vi "Main Tclk.vi"() -> ()   [LabVIEW 2018] (continued)
                            }
                          }
                          n5159 = Select(t="^delete" ("replace string (\"\")"), s=w4601, f="^keep" ("replace string (\"\")")) -> (s? t:f=w4605:string)
                          n5160 = Search and Replace String(input string=w4610, search string=":", replace string=w4611) -> (result string=w4607:string)  [unwired: 5 in, 3 out]
                          n5161 = Concatenate Strings(w4602, "^" ("string"), w4607, w4605) -> (w4616:string)
                          n5162 = Build Path(base path=w4615, name or relative path=w4616) -> (appended path=w4617:path)
                          n5163 = Open/Create/Replace File(file path (use dialog)=w4617, operation (0:open)=T49."replace or create") -> (refnum out=w4620:refnum<file>, error out=w4622:errorcluster)  [unwired: 1 in, 4 out]
                          n5164 = Close File(refnum=w4620, error in=w4622) -> (error out=w4621:errorcluster)  [unwired: 1 out]
                          n5165 = call <vilib>:"General Error Handler.vi"("type of dialog (OK msg:1)"=w4619, "error in (no error)"=w4621) -> ()  [unwired: 1 in, 13 out]
                        }
                      }
                      frame True {
                      }
                    }
                  }
                }
              }
            }
          }
          event "Delta X log": Mouse Down {
            n5166 = event-data() -> ("Coords"=w4639:T22)  [unwired: 8 out]
            n5167 = Unbundle By Name(w4639) -> ("Horizontal"=w4638:i32, "Vertical"=w4633:i32)
            n5168 = In Range and Coerce(upper limit=1200, x=w4638, lower limit=660 ("upper limit")) -> (In Range?=w4632:bool)  [unwired: 1 out]
            n5169 = In Range and Coerce(upper limit=510, x=w4633, lower limit=378 ("upper limit")) -> (In Range?=w4631:bool)  [unwired: 1 out]
            n5170 = And(x=w4632, y=w4631) -> (x .and. y?=w4630:bool)
            n5171 = case shown="True" w4630 {
              frame False {
              }
              frame True {
                n5172 = local read "Delta X toggle"() -> (w4640:bool)
                n5173 = case shown="False" w4640 {
                  frame False {
                    n5174 = local read "Log time array"() -> (w4643:u32[])
                    n5175 = local read "Delta X array"() -> (w4648:sgl[])
                    n5176 = local read "Delta X stop limit array"() -> (w4641:sgl[])
                    n5177 = local write "Delta X toggle"(TRUE ("Delta X toggle")) -> ()
                    n5178 = property on="Delta X log" class="XYGraph (strict)"("YScale.NameLbl.Text"="Delta X (nm)" ("Y Scale.Unit Label.Text")) -> ()  [unwired: 2 in, 2 out]
                    n5179 = Negate(x=w4641) -> (-x=w4644:sgl[])
                    n5180 = Bundle("Log time array"=w4643, "Delta X array"=w4648) -> (w4647:T83)  [unwired: 1 in]
                    n5181 = Bundle("Log time array"=w4643, "Delta X stop limit array"=w4641) -> (w4646:T84)  [unwired: 1 in]
                    n5182 = Bundle("Log time array"=w4643, w4644) -> (w4642:cluster{"Log time array":u32[], sgl[]})  [unwired: 1 in]
                    n5183 = Build Array(w4647, w4646, w4642) -> (w4645:T39)
                    n5184 = local write "Delta X log"(w4645) -> ()
                  }
                  frame True {
                    n5185 = local read "Log time array"() -> (w4651:u32[])
                    n5186 = local read "Delta X sum array"() -> (w4652:sgl[])
                    n5187 = local write "Delta X toggle"(FALSE ("Delta X toggle")) -> ()
                    n5188 = property on="Delta X log" class="XYGraph (strict)"("YScale.NameLbl.Text"="Delta X sum (nm)" ("Y Scale.Unit Label.Text")) -> ()  [unwired: 2 in, 2 out]
                    n5189 = Bundle("Log time array"=w4651, "Delta X sum array"=w4652) -> (w4654:T85)  [unwired: 1 in]
                    n5190 = Build Array(w4654) -> (w4653:T86)
                    n5191 = local write "Delta X log"(w4653) -> ()
                  }
                }
              }
            }
          }
          event "Delta Y log": Mouse Down {
            n5192 = event-data() -> ("Coords"=w4657:T22)  [unwired: 8 out]
            n5193 = Unbundle By Name(w4657) -> ("Horizontal"=w4666:i32, "Vertical"=w4661:i32)
            n5194 = In Range and Coerce(upper limit=1200, x=w4666, lower limit=660 ("upper limit")) -> (In Range?=w4660:bool)  [unwired: 1 out]
            n5195 = In Range and Coerce(upper limit=654, x=w4661, lower limit=522 ("upper limit")) -> (In Range?=w4659:bool)  [unwired: 1 out]
            n5196 = And(x=w4660, y=w4659) -> (x .and. y?=w4658:bool)
            n5197 = case shown="True" w4658 {
              frame False {
              }
              frame True {
                n5198 = local read "Delta Y toggle"() -> (w4667:bool)
                n5199 = case shown="True" w4667 {
                  frame False {
                    n5200 = local read "Log time array"() -> (w4672:u32[])
                    n5201 = local read "Delta Y array"() -> (w4674:sgl[])
                    n5202 = local read "Delta X stop limit array"() -> (w4668:sgl[])
                    n5203 = local write "Delta Y toggle"(TRUE ("Delta X toggle")) -> ()
                    n5204 = property on="Delta Y log" class="XYGraph (strict)"("YScale.NameLbl.Text"="Delta Y (nm)" ("Y Scale.Unit Label.Text")) -> ()  [unwired: 2 in, 2 out]
                    n5205 = Negate(x=w4668) -> (-x=w4671:sgl[])
                    n5206 = Bundle("Log time array"=w4672, "Delta Y array"=w4674) -> (w4669:T87)  [unwired: 1 in]
                    n5207 = Bundle("Log time array"=w4672, "Delta X stop limit array"=w4668) -> (w4670:T84)  [unwired: 1 in]
                    n5208 = Bundle("Log time array"=w4672, w4671) -> (w4673:cluster{"Log time array":u32[], sgl[]})  [unwired: 1 in]
                    n5209 = Build Array(w4669, w4670, w4673) -> (w4675:T39)
                    n5210 = local write "Delta Y log"(w4675) -> ()
                  }
                  frame True {
                    n5211 = local read "Log time array"() -> (w4679:u32[])
                    n5212 = local read "Delta Y sum array"() -> (w4680:sgl[])
                    n5213 = local write "Delta Y toggle"(FALSE ("Delta X toggle")) -> ()
                    n5214 = property on="Delta Y log" class="XYGraph (strict)"("YScale.NameLbl.Text"="Delta Y sum (nm)" ("Y Scale.Unit Label.Text")) -> ()  [unwired: 2 in, 2 out]
                    n5215 = Bundle("Log time array"=w4679, "Delta Y sum array"=w4680) -> (w4678:T88)  [unwired: 1 in]
                    n5216 = Build Array(w4678) -> (w4681:T89)
                    n5217 = local write "Delta Y log"(w4681) -> ()
                  }
                }
              }
            }
          }
          event "Delta Z log": Mouse Down {
            n5218 = event-data() -> ("Coords"=w4686:T22, "PlatMods"=w4685:T77)  [unwired: 7 out]
            n5219 = Unbundle By Name(w4686) -> ("Horizontal"=w4695:i32, "Vertical"=w4690:i32)
            n5220 = Unbundle By Name(w4685) -> ("Shift"=w4684:bool)
            n5221 = In Range and Coerce(upper limit=1200, x=w4695, lower limit=660 ("upper limit")) -> (In Range?=w4689:bool)  [unwired: 1 out]
            n5222 = In Range and Coerce(upper limit=798, x=w4690, lower limit=666 ("upper limit")) -> (In Range?=w4688:bool)  [unwired: 1 out]
            n5223 = And(x=w4689, y=w4688) -> (x .and. y?=w4687:bool)
            n5224 = case shown="True" w4687 {
              tunnel: w4684 -> [_ w4696]
              frame False {
              }
              frame True {
                n5225 = local read "Delta Z mode"() -> (w4706:u8)
                n5226 = case shown="1" w4706 {
                  tunnel: [w4709 w4716 w4748] -> w4700
                  tunnel: w4696 -> [_ w4715 _]
                  frame 0, Default {
                    n5227 = local read "Delta Z mode"() -> (w4712:u8)
                    n5228 = local read "Log time array"() -> (w4714:u32[])
                    n5229 = local read "Delta Z array"() -> (w4709:sgl[])
                    n5230 = Increment(x=w4712) -> (x+1=w4711:u8)
                    n5231 = property on="Delta Z log" class="XYGraph (strict)"("YScale.NameLbl.Text"="Delta Z (nm)" ("Y Scale.Unit Label.Text")) -> ()  [unwired: 2 in, 2 out]
                    n5232 = Bundle("Log time array"=w4714, "Delta Z array"=w4709) -> (w4713:T90)  [unwired: 1 in]
                    n5233 = local write "Delta Z mode"(w4711) -> ()
                    n5234 = local write "Delta Z log"(w4713) -> ()
                  }
                  frame 1 {
                    n5235 = case shown="True" w4715 {
                      tunnel: [w4717 w4723] -> w4716
                      frame False {
                        n5236 = local read "Log time array"() -> (w4722:u32[])
                        n5237 = local read "Milling Z voltage array"() -> (w4717:sgl[])
                        n5238 = local read "Delta Z mode"() -> (w4720:u8)
                        n5239 = Increment(x=w4720) -> (x+1=w4719:u8)
                        n5240 = property on="Delta Z log" class="XYGraph (strict)"("YScale.NameLbl.Text"="Milling Z Voltage (V)" ("Y Scale.Unit Label.Text")) -> ()  [unwired: 2 in, 2 out]
                        n5241 = Bundle("Log time array"=w4722, "Milling Z voltage array"=w4717) -> (w4721:T91)  [unwired: 1 in]
                        n5242 = local write "Delta Z mode"(w4719) -> ()
                        n5243 = local write "Delta Z log"(w4721) -> ()
                      }
                      frame True {
                        n5244 = local read "Milling Z voltage array"() -> (w4735:sgl[])
                        n5245 = Array Size(array=w4735) -> (size(s)=w4734:i32)
                        n5246 = for {
                          N: w4734 -> [_]
                          tunnel: w4735 -> [w4746]
                          tunnel: [w4738] -> w4732 mode=indexing
                          tunnel: 100 ("sample length") -> [w4742]
                          i -> [w4741]
                          n5247 = Increment(x=w4741) -> (x+1=w4737:i32)
                          n5248 = Subtract(x=w4737, y=w4742) -> (x-y=w4745:i32)
                          n5249 = Max & Min(x=w4742, y=w4737) -> (min(x,y)=w4740:i32)  [unwired: 1 out]
                          n5250 = Array Subset(array=w4746, index=w4745, length=w4740) -> (w4744:sgl[])
                          n5251 = for {
                            N: w4740 -> [_]
                            tunnel: [w4747] -> w4739 mode=indexing
                            i -> [w4747]
                          }
                          n5252 = call <vilib>:"Linear Fit.vi"("Y"=w4744, "X"=w4739) -> ("slope"=w4743:dbl)  [unwired: 9 in, 4 out]
                          n5253 = To Single Precision Float(number=w4743) -> (single precision float=w4738:sgl)
                        }
                        n5254 = local read "FIB Scan Parameters"() -> (w4733:T32)
                        n5255 = local read "Milling para"() -> (w4730:T35)
                        n5256 = Unbundle By Name(w4733) -> ("Z size (V)"=w4731:dbl)
                        n5257 = Unbundle By Name(w4730) -> ("FIB FOV (um)"=w4728:sgl)
                        n5258 = To Single Precision Float(number=w4731) -> (single precision float=w4726:sgl)
                        n5259 = local read "Log time array"() -> (w4725:u32[])
                        n5260 = Divide(x=w4732, y=w4726) -> (x/y=w4729:sgl[])
                        n5261 = Compound Arithmetic op=MULTIPLY(w4729, w4728, sgl -1000.0 ("value")) -> (w4723:sgl[])
                        n5262 = Bundle("Log time array"=w4725, w4723) -> (w4724:cluster{"Log time array":u32[], sgl[]})  [unwired: 1 in]
                        n5263 = local write "Delta Z log"(w4724) -> ()
                      }
                    }
                  }
                  frame 2 {
                    n5264 = local read "Log time array"() -> (w4752:u32[])
                    n5265 = local read "Delta image array"() -> (w4748:sgl[])
                    n5266 = property on="Delta Z log" class="XYGraph (strict)"("YScale.NameLbl.Text"="Delta Image" ("Y Scale.Unit Label.Text")) -> ()  [unwired: 2 in, 2 out]
                    n5267 = Bundle("Log time array"=w4752, "Delta image array"=w4748) -> (w4751:T92)  [unwired: 1 in]
                    n5268 = local write "Delta Z mode"(u8 0 ("Delta Z mode")) -> ()
                    n5269 = local write "Delta Z log"(w4751) -> ()
                  }
                }
                n5270 = Array Subset(array=w4700, index=1) -> (w4699:sgl[])  [unwired: 1 in]
                n5271 = Array Size(array=w4699) -> (size(s)=w4697:i32)
                n5272 = call "Auto limits.vi"("Minimum half range"=0.2, "# of interquartile range or stdev"=1.5 ("# of sigma"), "Input array"=w4699) -> ("Low limit"=w4705:dbl, "High limit"=w4704:dbl)  [unwired: 6 in, 1 out]
                n5273 = Not Equal To 0?(x=w4697) -> (x != 0?=w4698:bool)
                n5274 = case shown="True" w4698 {
                  tunnel: w4704 -> [_ w4708]
                  tunnel: w4705 -> [_ w4707]
                  frame False {
                  }
                  frame True {
                    n5275 = property on="Delta Z log" class="XYGraph (strict)"("YScale.Maximum"=w4708) -> ()  [unwired: 2 in, 2 out]
                    n5276 = property on="Delta Z log" class="XYGraph (strict)"("YScale.Minimum"=w4707) -> ()  [unwired: 2 in, 2 out]
                  }
                }
              }
            }
          }
          event "Specimen I log": Mouse Down {
            n5277 = event-data() -> ("Coords"=w4754:T22)  [unwired: 8 out]
            n5278 = Unbundle By Name(w4754) -> ("Horizontal"=w4762:i32, "Vertical"=w4757:i32)
            n5279 = In Range and Coerce(upper limit=1200, x=w4762, lower limit=660 ("upper limit")) -> (In Range?=w4756:bool)  [unwired: 1 out]
            n5280 = In Range and Coerce(upper limit=654, x=w4757, lower limit=522 ("upper limit")) -> (In Range?=w4755:bool)  [unwired: 1 out]
            n5281 = And(x=w4756, y=w4755) -> (x .and. y?=w4753:bool)
            n5282 = case shown="True" w4753 {
              frame False {
              }
              frame True {
                n5283 = local read "Specimen current toggle"() -> (w4763:bool)
                n5284 = case shown="False" w4763 {
                  frame False {
                    n5285 = local read "Log time array"() -> (w4767:u32[])
                    n5286 = local read "Specimen I array"() -> (w4772:sgl[])
                    n5287 = local read "Specimen I high limit array"() -> (w4766:sgl[])
                    n5288 = local read "Specimen I low limit array"() -> (w4765:sgl[])
                    n5289 = property on="Specimen I log" class="XYGraph (strict)"("YScale.NameLbl.Text"="Specimen @ FIB (nA)" ("Y Scale.Unit Label.Text")) -> ()  [unwired: 2 in, 2 out]
                    n5290 = local write "Specimen current toggle"(TRUE ("Delta X toggle")) -> ()
                    n5291 = Bundle("Log time array"=w4767, "Specimen I array"=w4772) -> (w4769:T93)  [unwired: 1 in]
                    n5292 = Bundle("Log time array"=w4767, "Specimen I high limit array"=w4766) -> (w4770:T94)  [unwired: 1 in]
                    n5293 = Bundle("Log time array"=w4767, "Specimen I low limit array"=w4765) -> (w4764:T95)  [unwired: 1 in]
                    n5294 = Build Array(w4769, w4770, w4764) -> (w4768:T96)
                    n5295 = local write "Specimen I log"(w4768) -> ()
                  }
                  frame True {
                    n5296 = local read "Log time array"() -> (w4777:u32[])
                    n5297 = local read "SEM Specimen I array"() -> (w4781:sgl[])
                    n5298 = local read "SEM Specimen I high limit array"() -> (w4776:sgl[])
                    n5299 = local read "SEM Specimen I low limit array"() -> (w4775:sgl[])
                    n5300 = property on="Specimen I log" class="XYGraph (strict)"("YScale.NameLbl.Text"="Specimen @ SEM (nA)" ("Y Scale.Unit Label.Text")) -> ()  [unwired: 2 in, 2 out]
                    n5301 = local write "Specimen current toggle"(FALSE ("Delta X toggle")) -> ()
                    n5302 = Bundle("Log time array"=w4777, "SEM Specimen I array"=w4781) -> (w4779:T97)  [unwired: 1 in]
                    n5303 = Bundle("Log time array"=w4777, "SEM Specimen I high limit array"=w4776) -> (w4780:T98)  [unwired: 1 in]
                    n5304 = Bundle("Log time array"=w4777, "SEM Specimen I low limit array"=w4775) -> (w4774:T99)  [unwired: 1 in]
                    n5305 = Build Array(w4779, w4780, w4774) -> (w4778:T100)
                    n5306 = local write "Specimen I log"(w4778) -> ()
                  }
                }
              }
            }
          }
          event "Beam Dump log": Mouse Down {
            n5307 = event-data() -> ("Coords"=w4785:T22)  [unwired: 8 out]
            n5308 = Unbundle By Name(w4785) -> ("Horizontal"=w4793:i32, "Vertical"=w4788:i32)
            n5309 = In Range and Coerce(upper limit=1200, x=w4793, lower limit=660 ("upper limit")) -> (In Range?=w4787:bool)  [unwired: 1 out]
            n5310 = In Range and Coerce(upper limit=798, x=w4788, lower limit=666 ("upper limit")) -> (In Range?=w4786:bool)  [unwired: 1 out]
            n5311 = And(x=w4787, y=w4786) -> (x .and. y?=w4784:bool)
            n5312 = case shown="True" w4784 {
              frame False {
              }
              frame True {
                n5313 = local read "Beam dump display"() -> (w4794:u8)
                n5314 = case shown="2" w4794 {
                  frame 0, Default {
                    w4804 = u8 1 items=["B.D.1", "B.D.2", "Mill"] ("Beam dump display")
                    n5315 = local read "Log time array"() -> (w4801:u32[])
                    n5316 = local read "Beam Dump 2 array"() -> (w4803:sgl[])
                    n5317 = local read "BD2 high limit array"() -> (w4796:sgl[])
                    n5318 = local read "BD2 low limit array"() -> (w4795:sgl[])
                    n5319 = local write "Beam dump display"(w4804) -> ()
                    n5320 = property on="Beam Dump log" class="XYGraph (strict)"("YScale.NameLbl.Text"="Beam Dump 2 (nA)" ("Y Scale.Unit Label.Text")) -> ()  [unwired: 2 in, 2 out]
                    n5321 = Bundle("Log time array"=w4801, "Beam Dump 2 array"=w4803) -> (w4800:T101)  [unwired: 1 in]
                    n5322 = Bundle("Log time array"=w4801, "BD2 high limit array"=w4796) -> (w4799:T102)  [unwired: 1 in]
                    n5323 = Bundle("Log time array"=w4801, "BD2 low limit array"=w4795) -> (w4798:T103)  [unwired: 1 in]
                    n5324 = Build Array(w4800, w4799, w4798) -> (w4797:T104)
                    n5325 = local write "Beam Dump log"(w4797) -> ()
                  }
                  frame 1 {
                    w4812 = u8 2 items=["B.D.1", "B.D.2", "Mill"] ("Beam dump display")
                    n5326 = local read "Log time array"() -> (w4806:u32[])
                    n5327 = local read "Milling I array"() -> (w4814:sgl[])
                    n5328 = local read "Milling I high limit array"() -> (w4809:sgl[])
                    n5329 = local read "Milling I low limit array"() -> (w4808:sgl[])
                    n5330 = local write "Beam dump display"(w4812) -> ()
                    n5331 = property on="Beam Dump log" class="XYGraph (strict)"("YScale.NameLbl.Text"="Mill Current (nA)" ("Y Scale.Unit Label.Text")) -> ()  [unwired: 2 in, 2 out]
                    n5332 = Bundle("Log time array"=w4806, "Milling I array"=w4814) -> (w4807:T105)  [unwired: 1 in]
                    n5333 = Bundle("Log time array"=w4806, "Milling I high limit array"=w4809) -> (w4811:T106)  [unwired: 1 in]
                    n5334 = Bundle("Log time array"=w4806, "Milling I low limit array"=w4808) -> (w4810:T107)  [unwired: 1 in]
                    n5335 = Build Array(w4807, w4811, w4810) -> (w4805:T108)
                    n5336 = local write "Beam Dump log"(w4805) -> ()
                  }
                  frame 2 {
                    w4824 = u8 0 items=["B.D.1", "B.D.2", "Mill"] ("Beam dump display")
                    n5337 = local read "Log time array"() -> (w4816:u32[])
                    n5338 = local read "Beam Dump 1 array"() -> (w4823:sgl[])
                    n5339 = local read "BD1 high limit array"() -> (w4820:sgl[])
                    n5340 = local read "BD1 low limit array"() -> (w4819:sgl[])
                    n5341 = local write "Beam dump display"(w4824) -> ()
                    n5342 = property on="Beam Dump log" class="XYGraph (strict)"("YScale.NameLbl.Text"="Beam Dump 1 (nA)" ("Y Scale.Unit Label.Text")) -> ()  [unwired: 2 in, 2 out]
                    n5343 = Bundle("Log time array"=w4816, "Beam Dump 1 array"=w4823) -> (w4818:T109)  [unwired: 1 in]
                    n5344 = Bundle("Log time array"=w4816, "BD1 high limit array"=w4820) -> (w4817:T110)  [unwired: 1 in]
                    n5345 = Bundle("Log time array"=w4816, "BD1 low limit array"=w4819) -> (w4821:T111)  [unwired: 1 in]
                    n5346 = Build Array(w4818, w4817, w4821) -> (w4815:T112)
                    n5347 = local write "Beam Dump log"(w4815) -> ()
                  }
                }
              }
            }
          }
          event "Request to reheat": Value Change {
            n5348 = event-data() -> ("NewVal"=w4825:bool)  [unwired: 6 out]
            n5349 = case shown="True" w4825 {
              frame False {
              }
              frame True {
                n5350 = stacked-sequence {
                  frame #0 {
                    n5351 = Two Button Dialog(message="Reheat FIB source?") -> (T button?=w4826:bool)  [unwired: 2 in]
                    n5352 = local write "Start Reheat"(w4826) -> ()
                  }
                  frame #1 {
                    n5353 = local write "Request to reheat"(FALSE ("Request to reheat")) -> ()
                  }
                }
              }
            }
          }
          event "Request to stop reheat": Value Change {
            n5354 = event-data() -> ("NewVal"=w4829:bool)  [unwired: 6 out]
            n5355 = case shown="True" w4829 {
              frame False {
              }
              frame True {
                n5356 = stacked-sequence {
                  frame #0 {
                    n5357 = Two Button Dialog(message="Stop FIB Reheat?") -> (T button?=w4830:bool)  [unwired: 2 in]
                    n5358 = local write "Stop Reheat"(w4830) -> ()
                  }
                  frame #1 {
                    n5359 = local write "Request to stop reheat"(FALSE ("Request to reheat")) -> ()
                  }
                }
              }
            }
          }
          event "Open FIB gun valve": Value Change {
            n5360 = event-data() -> ("OldVal"=w4833:bool, "NewVal"=w4834:bool)  [unwired: 5 out]
            n5361 = case shown="True" w4834 {
              tunnel: w4833 -> [w4835 w4841]
              frame False {
                n5362 = stacked-sequence {
                  tunnel: w4835 -> [w4836 _]
                  frame #0 {
                    n5363 = local write "Open FIB gun valve"(w4836) -> ()
                  }
                  frame #1 {
                    n5364 = Two Button Dialog(message="Close FIB Gun Valve?") -> (T button?=w4837:bool)  [unwired: 2 in]
                    n5365 = case shown="True" w4837 {
                      frame False {
                      }
                      frame True {
                        n5366 = local read "Api"() -> (w4840:refnum<k7>)
                        n5367 = call "SmartSEM Remote API FIB Gun Valve.vi"("FIB Gun Valve"=enum16{"Close", "Open"}."Close", "Api"=w4840) -> ()  [unwired: 8 in, 2 out]
                      }
                    }
                  }
                }
              }
              frame True {
                n5368 = stacked-sequence {
                  tunnel: w4841 -> [w4842 _]
                  frame #0 {
                    n5369 = local write "Open FIB gun valve"(w4842) -> ()
                  }
                  frame #1 {
                    n5370 = Two Button Dialog(message="Open FIB Gun Valve?") -> (T button?=w4843:bool)  [unwired: 2 in]
                    n5371 = case shown="True" w4843 {
                      frame False {
                      }
                      frame True {
                        n5372 = local read "Api"() -> (w4846:refnum<k7>)
                        n5373 = call "SmartSEM Remote API FIB Gun Valve.vi"("FIB Gun Valve"=enum16{"Close", "Open"}."Open", "Api"=w4846) -> ()  [unwired: 8 in, 2 out]
                      }
                    }
                  }
                }
              }
            }
          }
          event "Turn on FIB gun": Value Change {
            n5374 = event-data() -> ("NewVal"=w4848:bool)  [unwired: 6 out]
            n5375 = local read "Machine Type"() -> (w4847:u8)
            n5376 = case shown="True" w4848 {
              tunnel: w4847 -> [_ w4849]
              frame False {
              }
              frame True {
                n5377 = case shown="2" w4849 {
                  frame 0 {
                    n5378 = stacked-sequence {
                      frame #0 {
                        n5379 = local read "HV Data Output"() -> (w4852:T18)
                        n5380 = Unbundle By Name(w4852) -> ("Tip Lifetime (hr)"=w4851:sgl)
                        n5381 = Equal To 0?(x=w4851) -> (x = 0?=w4850:bool)
                        n5382 = case shown="True" w4850 {
                          frame False {
                          }
                          frame True {
                            n5383 = for {
                              N: 5 -> [_]
                              stop <- w4855 stop-if-true
                              n5384 = Wait Until Next ms Multiple(millisecond multiple=u32 100) -> ()  [unwired: 1 out]
                              n5385 = call "Read FIB Log Files.vi"("Log file path"=path "C:/Program Files (x86)/FEI Company/BDS/LogHVData.log") -> ("HV Data Output"=w4872:T113)  [unwired: 9 in, 1 out]
                              n5386 = Unbundle By Name(w4872) -> ("Filament (A)"=w4871:sgl, "Acclerator (V)"=w4870:sgl, "AccI (uA)"=w4869:sgl, "Extractor (V)"=w4868:sgl, "Emission (uA)"=w4867:sgl, "Suppressor (V)"=w4866:sgl, "SuppI (uA)"=w4865:sgl, "Lens1 (V)"=w4864:sgl, "Lens1I (uA)"=w4863:sgl, "Lens2 (V)"=w4862:sgl, "Lens2I (uA)"=w4861:sgl, "Tip Lifetime (hr)"=w4858:sgl)
                              n5387 = local write "HV Data Output"(w4872) -> ()
                              n5388 = Build Array(w4871, w4870, w4869, w4868, w4867, w4866, w4865, w4864, w4863, w4862, w4861, w4858) -> (w4860:sgl[])
                              n5389 = Add Array Elements(numeric array=w4860) -> (sum=w4859:sgl)
                              n5390 = Not Equal To 0?(x=w4859) -> (x != 0?=w4856:bool)
                              n5391 = Not Equal To 0?(x=w4858) -> (x != 0?=w4857:bool)
                              n5392 = Or(x=w4856, y=w4857) -> (x .or. y?=w4855:bool)
                            }
                          }
                        }
                      }
                      frame #1 {
                        n5393 = Two Button Dialog(message="Turn FIB Gun on without Reheat?") -> (T button?=w4874:bool)  [unwired: 2 in]
                        "Turn FIB Gun on" <- w4874
                        n5394 = local write "Start Reheat"(w4874) -> ()
                      }
                      frame #2 {
                        n5395 = local write "Turn on FIB gun"(FALSE ("Request to reheat")) -> ()
                      }
                    }
                  }
                  frame 1, Default {
                  }
                  frame 2 {
                    n5396 = Two Button Dialog(message="Turn FIB Gun on without Reheat?") -> (T button?=w4877:bool)  [unwired: 2 in]
                    n5397 = case shown="True" w4877 {
                      frame False {
                      }
                      frame True {
                        n5398 = local read "Api"() -> (w4881:refnum<k7>)
                        n5399 = invoke class="_EMApi" method="Execute"(reference=w4881, "lpszCommand"="CMD_FIB_GUN_ON") -> ()  [unwired: 2 in, 4 out]
                        n5400 = property on="Turn off FIB gun" class="Bool (strict)"("DisabledEnum"=T44."Enabled" ("Disabled")) -> ()  [unwired: 2 in, 2 out]
                      }
                    }
                  }
                }
              }
            }
          }
          event "Turn off FIB gun": Value Change {
            n5401 = event-data() -> ("NewVal"=w4882:bool)  [unwired: 6 out]
            n5402 = case shown="True" w4882 {
              frame False {
              }
              frame True {
                n5403 = Two Button Dialog(message="Turn FIB Gun off?") -> (T button?=w4883:bool)  [unwired: 2 in]
                n5404 = case shown="True" w4883 {
                  frame False {
                    n5405 = local write "Turn off FIB gun"(FALSE ("Turn off FIB gun")) -> ()
                  }
                  frame True {
                    n5406 = local read "Api"() -> (w4887:refnum<k7>)
                    n5407 = invoke class="_EMApi" method="Execute"(reference=w4887, "lpszCommand"="CMD_FIB_GUN_OFF") -> ()  [unwired: 2 in, 4 out]
                  }
                }
              }
            }
          }
          event "Turn FIB gun standby": Value Change {
            n5408 = event-data() -> ("NewVal"=w4888:bool)  [unwired: 6 out]
            n5409 = case shown="True" w4888 {
              frame False {
              }
              frame True {
                n5410 = Two Button Dialog(message="Put FIB Gun to Standby?") -> (T button?=w4889:bool)  [unwired: 2 in]
                n5411 = case shown="True" w4889 {
                  frame False {
                    n5412 = local write "Turn FIB gun standby"(FALSE ("Turn off FIB gun")) -> ()
                  }
                  frame True {
                    n5413 = local read "Api"() -> (w4893:refnum<k7>)
                    n5414 = invoke class="_EMApi" method="Execute"(reference=w4893, "lpszCommand"="CMD_FIB_GUN_STANDBY") -> ()  [unwired: 2 in, 4 out]
                  }
                }
              }
            }
          }
          event "Get V/I slope": Value Change {
            n5415 = event-data() -> ("NewVal"=w4894:bool)  [unwired: 6 out]
            n5416 = case shown="True" w4894 {
              frame False {
              }
              frame True {
                n5417 = Two Button Dialog(message="Check FIB source V/I slope?") -> (T button?=w4895:bool)  [unwired: 2 in]
                n5418 = case shown="True" w4895 {
                  frame False {
                    n5419 = local write "Get V/I slope"(FALSE ("Turn off FIB gun")) -> ()
                  }
                  frame True {
                    n5420 = local read "Api"() -> (w4900:refnum<k7>)
                    n5421 = local write "Get V/I slope"(FALSE ("Turn off FIB gun")) -> ()
                    n5422 = call "SmartSEM Remote API FIB VI slope.vi"("Api"=w4900) -> ("V/I slope"=→"FIB V/I slope":sgl)  [unwired: 8 in, 2 out]
                  }
                }
              }
            }
          }
          event "Email Alert Recipients": Value Change {
            n5423 = event-data() -> ("NewVal"=w4902:string[])  [unwired: 6 out]
            n5424 = local read "FIB"() -> (w4901:bool)
            n5425 = case shown="True" w4901 {
              tunnel: w4902 -> [_ w4903]
              frame False {
              }
              frame True {
                n5426 = local read "Email recipents file"() -> (w4909:path)
                n5427 = Open/Create/Replace File(file path (use dialog)=w4909, operation (0:open)=T49."replace or create") -> (refnum out=w4908:refnum<file>, error out=w4907:errorcluster)  [unwired: 4 in, 1 out]
                n5428 = Write to Text File(file (use dialog)=w4908, text=w4903, error in=w4907) -> (refnum out=w4906:refnum<file>, error out=w4905:errorcluster)  [unwired: 1 in, 1 out]
                n5429 = Close File(refnum=w4906, error in=w4905) -> ()  [unwired: 2 out]
              }
            }
          }
          event "Focus Index Options.X Grids": Mouse Down; "Focus Index Options.X Grids": Value Change {
            n5430 = event-data() -> ()  [unwired: 5 out]
            n5431 = disable-structure shown="Disabled" {
              frame Disabled {
                n5432 = local read "Focus Index Options"() -> (w4922:T28)
                n5433 = Unbundle By Name(w4922) -> ("Focus Index primary grid center"=w4914:bool, "Primary X index"=w4923:u8[][], "Y Grids"=w4924:u8[][], "Primary Y index"=w4925:u8[][])  [unwired: 1 out]
                n5434 = local read "SEM Scan Parameters"() -> (w4930:T26)
                n5435 = Unbundle By Name(w4922) -> ("X Grids"=w4926:u8[][])
                n5436 = Unbundle By Name(w4930) -> ("X tiles"=w4929:u8, "Y tiles"=w4928:u8)
                n5437 = Select(t=2.0 ("Data Entry Limits:Increment"), s=w4914, f=1.0 ("Data Entry Limits:Increment")) -> (s? t:f=w4916:dbl)
                n5438 = call "2D array edit.vi"("min"=u8 1 ("x"), "max"=u8 100 ("x"), "Set boundaries"=TRUE ("Set boundary"), "Data Entry Limits:Increment"=w4916, "Display Format:Precision"=u8 0, "Rows"=w4928, "Columns"=w4929, "Caption.Text"="X Grids", "Input array"=w4926) -> ("Output array"=w4921:sgl[][])  [unwired: 2 in]
                n5439 = case shown="False" w4914 {
                  tunnel: w4921 -> [w4937 w4959]
                  tunnel: w4923 -> [w4936 _]
                  tunnel: w4924 -> [w4935 w4958]
                  tunnel: w4925 -> [w4934 _]
                  tunnel: w4922 -> [w4933 w4957]
                  frame False {
                    n5440 = for {
                      tunnel: w4937 -> [w4949] mode=indexing
                      tunnel: w4936 -> [w4948] mode=indexing
                      tunnel: [w4947] -> w4941 mode=indexing
                      tunnel: w4935 -> [w4946] mode=indexing
                      tunnel: w4934 -> [w4945] mode=indexing
                      tunnel: [w4944] -> w4940 mode=indexing
                      tunnel: u8 1 ("x") -> [w4943]
                      tunnel: [w4942] -> w4932 mode=indexing
                      n5441 = for {
                        tunnel: w4949 -> [w4950] mode=indexing
                        tunnel: w4948 -> [w4956] mode=indexing
                        tunnel: [w4955] -> w4947 mode=indexing
                        tunnel: w4946 -> [w4954] mode=indexing
                        tunnel: w4945 -> [w4953] mode=indexing
                        tunnel: [w4952] -> w4944 mode=indexing
                        tunnel: w4943 -> [w4951]
                        tunnel: [w4950] -> w4942 mode=indexing
                        n5442 = In Range and Coerce(upper limit=w4950, x=w4956, lower limit=w4951) -> (coerced(x)=w4955:sgl)  [unwired: 1 out]
                        n5443 = In Range and Coerce(upper limit=w4954, x=w4953, lower limit=w4951) -> (coerced(x)=w4952:u8)  [unwired: 1 out]
                      }
                    }
                    n5444 = Bundle By Name(cluster=w4933, "X Grids"=w4932, "Primary X index"=w4941, "Primary Y index"=w4940) -> (w4939:T28)
                    n5445 = local write "Focus Index Options"(w4939) -> ()
                  }
                  frame True {
                    n5446 = for {
                      tunnel: w4959 -> [w4970] mode=indexing
                      tunnel: w4958 -> [w4969] mode=indexing
                      tunnel: [w4968] -> w4963 mode=indexing
                      tunnel: [w4967] -> w4962 mode=indexing
                      tunnel: [w4966] -> w4961 mode=indexing
                      tunnel: [w4965] -> w4960 mode=indexing
                      n5447 = for {
                        tunnel: w4970 -> [w4976] mode=indexing
                        tunnel: w4969 -> [w4975] mode=indexing
                        tunnel: [w4974] -> w4968 mode=indexing
                        tunnel: [w4973] -> w4967 mode=indexing
                        tunnel: [w4972] -> w4966 mode=indexing
                        tunnel: [w4971] -> w4965 mode=indexing
                        n5448 = To Single Precision Float(number=w4976) -> (single precision float=w4979:sgl)
                        n5449 = To Single Precision Float(number=w4975) -> (single precision float=w4978:sgl)
                        n5450 = expression code="x/2"(w4979) -> (w4980:sgl)
                        n5451 = expression code="x/2"(w4978) -> (w4977:sgl)
                        n5452 = Round Toward +Infinity(x=w4980) -> (ceil(x): smallest int >= x=w4973:sgl)
                        n5453 = Round Toward +Infinity(x=w4977) -> (ceil(x): smallest int >= x=w4971:sgl)
                        n5454 = expression code="x*2-1"(w4973) -> (w4974:sgl)
                        n5455 = expression code="x*2-1"(w4971) -> (w4972:sgl)
                      }
                    }
                    n5456 = Bundle By Name(cluster=w4957, "X Grids"=w4963, "Primary X index"=w4962, "Y Grids"=w4961, "Primary Y index"=w4960) -> (w4964:T28)
                    n5457 = local write "Focus Index Options"(w4964) -> ()
                  }
                }
              }
              frame Enabled {
              }
            }
            n5458 = local write "FI array for stop limit"(sgl[] [] ("FI array for stop limit")) -> ()
            n5459 = local read "Focus Index Options"() -> (w4910:T28)
            n5460 = local read "SEM Scan Parameters"() -> (w4911:T26)
            n5461 = call "Focus Grid Chooser.vi"("SEM Scan Parameters"=w4911, "Focus Index Options"=w4910) -> ("Focus Index Options Out"=w4912:T28)  [unwired: 9 in]
            n5462 = local write "Focus Index Options"(w4912) -> ()
          }
          event "Focus Index Options.Y Grids": Mouse Down; "Focus Index Options.Y Grids": Value Change {
            n5463 = event-data() -> ()  [unwired: 5 out]
            n5464 = disable-structure shown="Disabled" {
              frame Disabled {
                n5465 = local read "Focus Index Options"() -> (w4994:T28)
                n5466 = Unbundle By Name(w4994) -> ("Focus Index primary grid center"=w4987:bool, "X Grids"=w4986:u8[][], "Primary X index"=w4995:u8[][], "Primary Y index"=w4996:u8[][])  [unwired: 1 out]
                n5467 = local read "SEM Scan Parameters"() -> (w5001:T26)
                n5468 = Unbundle By Name(w4994) -> ("Y Grids"=w4997:u8[][])
                n5469 = Unbundle By Name(w5001) -> ("X tiles"=w5000:u8, "Y tiles"=w4999:u8)
                n5470 = Select(t=2.0 ("Data Entry Limits:Increment"), s=w4987, f=1.0 ("Data Entry Limits:Increment")) -> (s? t:f=w4989:dbl)
                n5471 = call "2D array edit.vi"("min"=u8 1 ("x"), "max"=u8 100 ("x"), "Set boundaries"=TRUE ("Set boundary"), "Data Entry Limits:Increment"=w4989, "Display Format:Precision"=u8 0, "Rows"=w4999, "Columns"=w5000, "Caption.Text"="Y Grids", "Input array"=w4997) -> ("Output array"=w4985:sgl[][])  [unwired: 2 in]
                n5472 = case shown="False" w4987 {
                  tunnel: w4986 -> [w5008 w5030]
                  tunnel: w4995 -> [w5007 _]
                  tunnel: w4985 -> [w5006 w5029]
                  tunnel: w4996 -> [w5005 _]
                  tunnel: w4994 -> [w5004 w5028]
                  frame False {
                    n5473 = for {
                      tunnel: w5008 -> [w5020] mode=indexing
                      tunnel: w5007 -> [w5019] mode=indexing
                      tunnel: [w5018] -> w5012 mode=indexing
                      tunnel: w5006 -> [w5017] mode=indexing
                      tunnel: w5005 -> [w5016] mode=indexing
                      tunnel: [w5015] -> w5011 mode=indexing
                      tunnel: u8 1 ("x") -> [w5014]
                      tunnel: [w5013] -> w5003 mode=indexing
                      n5474 = for {
                        tunnel: w5020 -> [w5027] mode=indexing
                        tunnel: w5019 -> [w5026] mode=indexing
                        tunnel: [w5025] -> w5018 mode=indexing
                        tunnel: w5017 -> [w5021] mode=indexing
                        tunnel: w5016 -> [w5024] mode=indexing
                        tunnel: [w5023] -> w5015 mode=indexing
                        tunnel: w5014 -> [w5022]
                        tunnel: [w5021] -> w5013 mode=indexing
                        n5475 = In Range and Coerce(upper limit=w5027, x=w5026, lower limit=w5022) -> (coerced(x)=w5025:u8)  [unwired: 1 out]
                        n5476 = In Range and Coerce(upper limit=w5021, x=w5024, lower limit=w5022) -> (coerced(x)=w5023:sgl)  [unwired: 1 out]
                      }
                    }
                    n5477 = Bundle By Name(cluster=w5004, "Primary X index"=w5012, "Y Grids"=w5003, "Primary Y index"=w5011) -> (w5010:T28)
                    n5478 = local write "Focus Index Options"(w5010) -> ()
                  }
                  frame True {
                    n5479 = for {
                      tunnel: w5030 -> [w5041] mode=indexing
                      tunnel: w5029 -> [w5040] mode=indexing
                      tunnel: [w5039] -> w5034 mode=indexing
                      tunnel: [w5038] -> w5033 mode=indexing
                      tunnel: [w5037] -> w5032 mode=indexing
                      tunnel: [w5036] -> w5031 mode=indexing
                      n5480 = for {
                        tunnel: w5041 -> [w5047] mode=indexing
                        tunnel: w5040 -> [w5046] mode=indexing
                        tunnel: [w5045] -> w5039 mode=indexing
                        tunnel: [w5044] -> w5038 mode=indexing
                        tunnel: [w5043] -> w5037 mode=indexing
                        tunnel: [w5042] -> w5036 mode=indexing
                        n5481 = To Single Precision Float(number=w5047) -> (single precision float=w5050:sgl)
                        n5482 = To Single Precision Float(number=w5046) -> (single precision float=w5049:sgl)
                        n5483 = expression code="x/2"(w5050) -> (w5051:sgl)
                        n5484 = expression code="x/2"(w5049) -> (w5048:sgl)
                        n5485 = Round Toward +Infinity(x=w5051) -> (ceil(x): smallest int >= x=w5044:sgl)
                        n5486 = Round Toward +Infinity(x=w5048) -> (ceil(x): smallest int >= x=w5042:sgl)
                        n5487 = expression code="x*2-1"(w5044) -> (w5045:sgl)
                        n5488 = expression code="x*2-1"(w5042) -> (w5043:sgl)
                      }
                    }
                    n5489 = Bundle By Name(cluster=w5028, "X Grids"=w5034, "Primary X index"=w5033, "Y Grids"=w5032, "Primary Y index"=w5031) -> (w5035:T28)
                    n5490 = local write "Focus Index Options"(w5035) -> ()
                  }
                }
              }
              frame Enabled {
              }
            }
            n5491 = local write "FI array for stop limit"(sgl[] [] ("FI array for stop limit")) -> ()
            n5492 = local read "Focus Index Options"() -> (w4981:T28)
            n5493 = local read "SEM Scan Parameters"() -> (w4982:T26)
            n5494 = call "Focus Grid Chooser.vi"("SEM Scan Parameters"=w4982, "Focus Index Options"=w4981) -> ("Focus Index Options Out"=w4983:T28)  [unwired: 9 in]
            n5495 = local write "Focus Index Options"(w4983) -> ()
          }
          event "Focus Index Options.Primary X index": Mouse Down; "Focus Index Options.Primary X index": Value Change {
            n5496 = event-data() -> ()  [unwired: 5 out]
            n5497 = disable-structure shown="Disabled" {
              frame Disabled {
                n5498 = local read "Focus Index Options"() -> (w5060:T28)
                n5499 = Unbundle By Name(w5060) -> ("Focus Index primary grid center"=w5065:bool, "X Grids"=w5064:u8[][], "Primary X index"=w5063:u8[][])
                n5500 = local read "SEM Scan Parameters"() -> (w5071:T26)
                n5501 = case shown="True" w5065 {
                  tunnel: w5064 -> [w5075 _]
                  tunnel: w5063 -> [_ w5081]
                  tunnel: [1.0 ("Data Entry Limits:Increment") 0.0 ("Data Entry Limits:Increment")] -> w5062
                  tunnel: [u8 1 ("x") w5079] -> w5058
                  tunnel: [w5074 w5080] -> w5057
                  tunnel: [T44."Enabled" ("Disabled") T44."Disabled and Grayed Out" ("Disabled")] -> w5056
                  frame False {
                    n5502 = Array Max & Min(array=w5075) -> (max value=w5074:u8)  [unwired: 3 out]
                  }
                  frame True {
                    n5503 = Array Max & Min(array=w5081) -> (max value=w5080:u8, min value=w5079:u8)  [unwired: 2 out]
                  }
                }
                n5504 = Unbundle By Name(w5060) -> ("Primary X index"=w5067:u8[][])
                n5505 = Unbundle By Name(w5071) -> ("X tiles"=w5070:u8, "Y tiles"=w5069:u8)
                n5506 = call "2D array edit.vi"("min"=w5058, "max"=w5057, "Set boundaries"=TRUE ("Set boundary"), "Disabled"=w5056, "Data Entry Limits:Increment"=w5062, "Display Format:Precision"=u8 0, "Rows"=w5069, "Columns"=w5070, "Caption.Text"="Primary X grid", "Input array"=w5067) -> ("Output array"=w5061:sgl[][])  [unwired: 1 in]
                n5507 = Bundle By Name(cluster=w5060, "Primary X index"=w5061) -> (w5059:T28)
                n5508 = local write "Focus Index Options"(w5059) -> ()
              }
              frame Enabled {
              }
            }
            n5509 = local write "FI array for stop limit"(sgl[] [] ("FI array for stop limit")) -> ()
            n5510 = local read "Focus Index Options"() -> (w5052:T28)
            n5511 = local read "SEM Scan Parameters"() -> (w5053:T26)
            n5512 = call "Focus Grid Chooser.vi"("SEM Scan Parameters"=w5053, "Focus Index Options"=w5052) -> ("Focus Index Options Out"=w5054:T28)  [unwired: 9 in]
            n5513 = local write "Focus Index Options"(w5054) -> ()
          }
          event "Focus Index Options.Primary Y index": Mouse Down; "Focus Index Options.Primary Y index": Value Change {
            n5514 = event-data() -> ()  [unwired: 5 out]
            n5515 = disable-structure shown="Disabled" {
              frame Disabled {
                n5516 = local read "Focus Index Options"() -> (w5091:T28)
                n5517 = Unbundle By Name(w5091) -> ("Focus Index primary grid center"=w5096:bool, "Y Grids"=w5095:u8[][], "Primary Y index"=w5094:u8[][])
                n5518 = local read "SEM Scan Parameters"() -> (w5102:T26)
                n5519 = case shown="False" w5096 {
                  tunnel: w5095 -> [w5106 _]
                  tunnel: w5094 -> [_ w5112]
                  tunnel: [1.0 ("Data Entry Limits:Increment") 0.0 ("Data Entry Limits:Increment")] -> w5093
                  tunnel: [u8 1 ("x") w5110] -> w5089
                  tunnel: [w5105 w5111] -> w5088
                  tunnel: [T44."Enabled" ("Disabled") T44."Disabled and Grayed Out" ("Disabled")] -> w5087
                  frame False {
                    n5520 = Array Max & Min(array=w5106) -> (max value=w5105:u8)  [unwired: 3 out]
                  }
                  frame True {
                    n5521 = Array Max & Min(array=w5112) -> (max value=w5111:u8, min value=w5110:u8)  [unwired: 2 out]
                  }
                }
                n5522 = Unbundle By Name(w5091) -> ("Primary Y index"=w5098:u8[][])
                n5523 = Unbundle By Name(w5102) -> ("X tiles"=w5101:u8, "Y tiles"=w5100:u8)
                n5524 = call "2D array edit.vi"("min"=w5089, "max"=w5088, "Set boundaries"=TRUE ("Set boundary"), "Disabled"=w5087, "Data Entry Limits:Increment"=w5093, "Display Format:Precision"=u8 0, "Rows"=w5100, "Columns"=w5101, "Caption.Text"="Primary Y grid", "Input array"=w5098) -> ("Output array"=w5092:sgl[][])  [unwired: 1 in]
                n5525 = Bundle By Name(cluster=w5091, "Primary Y index"=w5092) -> (w5090:T28)
                n5526 = local write "Focus Index Options"(w5090) -> ()
              }
              frame Enabled {
              }
            }
            n5527 = local write "FI array for stop limit"(sgl[] [] ("FI array for stop limit")) -> ()
            n5528 = local read "Focus Index Options"() -> (w5083:T28)
            n5529 = local read "SEM Scan Parameters"() -> (w5084:T26)
            n5530 = call "Focus Grid Chooser.vi"("SEM Scan Parameters"=w5084, "Focus Index Options"=w5083) -> ("Focus Index Options Out"=w5085:T28)  [unwired: 9 in]
            n5531 = local write "Focus Index Options"(w5085) -> ()
          }
          event "Det A": Mouse Down {
            n5532 = event-data() -> ()  [unwired: 9 out]
            n5533 = local read "Focus Index tiled"() -> (w5115:sgl[][])
            n5534 = local read "SEM Scan Parameters"() -> (w5119:T26)
            n5535 = Unbundle By Name(w5119) -> ("X tiles"=w5118:u8, "Y tiles"=w5117:u8)
